vi "overlay_generation.vi"(5 "center radius":dbl, 6 "Color":u32(colorbox)=16448250, 7 "number of rings":i32) -> (2 "Image Out":T1)   [LabVIEW 2011]
doc: "Creates Overlay pattern to help with the alignment of the setup. The input image is copied and a new memory space is create to hold the overlay image in order to keep the originally created pattern."
uses:
  <vilib>/vision/Image Controls.llb/IMAQ Image.ctl
  global_vars.vi
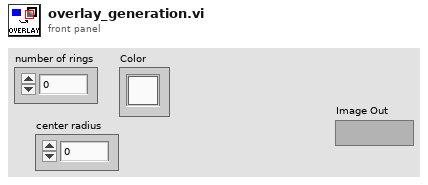
[diagram p1: front panel]
types:
  T1 = typedef "IMAQ Image.ctl" = refnum<image>
  T2 = cluster{"Desired Font (Application)":enum16{"User-specified Font", "Application Font", "System Font", "Dialog Font"}, "[User-specified Font]":cluster{"Font Name":string, "Size":i16, "Strikeout?":bool, "Italic?":bool, "Underline?":bool, "Outline?":bool, "Shadow?":bool, "Bold?":bool, "Rotation Angle":dbl}, "Horizontal Alignment":i16, "Vertical Alignment":i16}
  T3 = cluster{"Numeric Control":dbl, "Numeric Control":dbl, "Numeric Control":dbl, "Numeric Control":dbl}
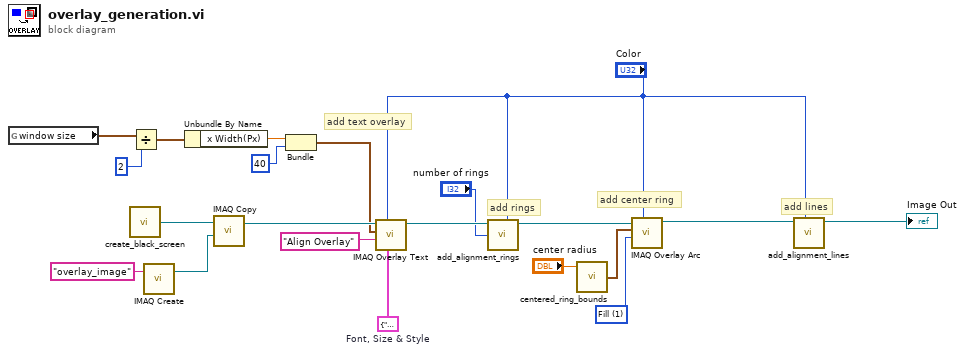
[diagram p0: block diagram]
diagram:
  w3 = u32 1 items=["Frame", "Fill"] ("Drawing Mode (Frame)")
  w20 = T2 {"Desired Font (Application)"=enum."User-specified Font", "[User-specified Font]"={"Font Name"="Arial", "Size"=30, "Strikeout?"=FALSE, "Italic?"=FALSE, "Underline?"=FALSE, "Outline?"=FALSE, "Shadow?"=FALSE, "Bold?"=TRUE, "Rotation Angle"=0.0}, "Horizontal Alignment"=1, "Vertical Alignment"=2}  # Font, Size & Style
  # "add lines"
  # "add center ring"
  # "add rings"
  # "add text overlay"
  n1 = global read "global_vars.vi" "window size"() -> (w13:cluster{"x Width(Px)":i32, "y height(Px)":i32})
  n2 = call "create_black_screen.vi"() -> ("img_black_screen"=w1:T1)  [unwired: 5 in]
  n3 = Divide(x=w13, y=2 ("y height(Px)")) -> (x/y=w12:cluster{"x Width(Px)":dbl, "y height(Px)":dbl})
  n4 = call "IMAQ Create"("Image Name"="overlay_image") -> ("New Image"=w17:T1)  [unwired: 4 in, 1 out]
  n5 = Unbundle By Name(w12) -> ("x Width(Px)"=w11:dbl)
  n6 = call "IMAQ Copy"("Image Dst"=w17, "Image Src"=w1) -> ("Image Dst Out"=w18:T1)  [unwired: 4 in, 1 out]
  n7 = Bundle("x Width(Px)"=w11, 40) -> (w16:cluster{"x Width(Px)":dbl, i32})  [unwired: 1 in]
  n8 = call "IMAQ Overlay Text"("Text Color (black)"="Color", "Font, Size & Style"=w20, "String"="Align Overlay", "Origin"=w16, "Image"=w18) -> ("Image Out"=w9:T1)  [unwired: 5 in, 1 out]
  n9 = call "add_alignment_rings.vi"("Color"="Color", "number of rings"="number of rings", "Image in"=w9) -> ("Image Out"=w5:T1)  [unwired: 6 in]
  n10 = call "centered_ring_bounds.vi"("radius R"="center radius") -> ("Bounding Rectangle"=w7:T3)  [unwired: 4 in]
  n11 = call "IMAQ Overlay Arc"("Color"="Color", "Drawing Mode (Frame)"=w3, "Bounding Rectangle"=w7, "Image"=w5) -> ("Image Out"=w4:T1)  [unwired: 6 in, 1 out]
  n12 = call "add_alignment_lines.vi"("Color"="Color", "Image in"=w4) -> ("Image out"=→"Image Out":T1)  [unwired: 9 in]
